vi "EditorPDF setPDFList.vi"(8 "error in (no error)":errorcluster, 11 "CreatePDF in":refnum<class "CreatePDF.lvclass">) -> (0 "error out":errorcluster, 3 "CreatePDF out":refnum<class "CreatePDF.lvclass">)   [LabVIEW 2018, in "CreatePDF.lvclass"]
uses:
  CreatePDF.lvclass
  <vilib>/Simplicity AI/SAI_PDF_API/Classes/Context/Controls/SAI_PDF_Text Align.ctl
  <vilib>/Simplicity AI/SAI_PDF_API/Classes/Context/Controls/SAI_PDF_Table Settings.ctl
  <vilib>/Simplicity AI/SAI_PDF_API/Classes/Context/Controls/SAI_PDF_Table Parameters.ctl
  <vilib>/Simplicity AI/SAI_PDF_API/Classes/Table Builder/Controls/SAI_PDF_Table Cell Alignment.ctl
  <vilib>/Simplicity AI/SAI_PDF_API/Classes/Context/Controls/SAI_PDF_Vertical Align.ctl
  CreatePDF.lvclass/CreatePDF.ctl
  <vilib>/Simplicity AI/SAI_PDF_API/Classes/Context/Methods/Public/Low Level/Add/SAI_PDF_Add Paragraph.vi
  <vilib>/Simplicity AI/SAI_PDF_API/Classes/Context/Context.lvclass
  <vilib>/Simplicity AI/SAI_PDF_API/Classes/Table Builder/Table Builder.lvclass
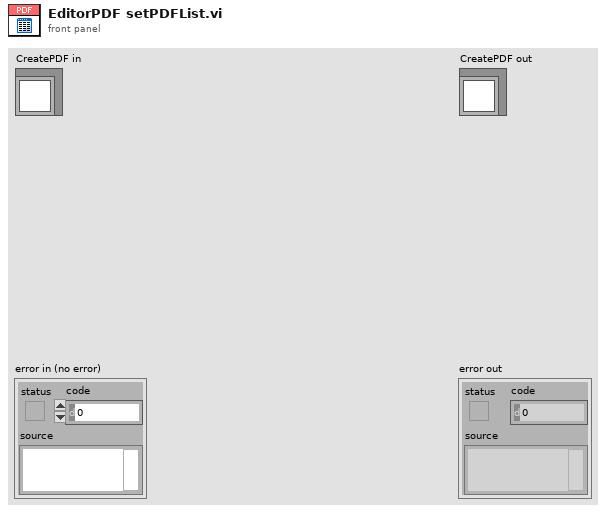
[diagram p1: front panel]
types:
  T1 = typedef "SAI_PDF_Toolkit.lvlib/Context.lvclass/SAI_PDF_Table Settings.ctl" = cluster{"Column Widths":sgl[], "Parameters":T2, "Cell Alignment":T3}
  T2 = typedef "SAI_PDF_Toolkit.lvlib/Context.lvclass/SAI_PDF_Table Parameters.ctl" = cluster{"Show Header":bool, "Background Colour":u32, "Colour Alternate Lines":bool, "Min Row Height":sgl, "Border Width":sgl}
  T3 = typedef "SAI_PDF_Toolkit.lvlib/Table Builder.lvclass/SAI_PDF_Table Cell Alignment.ctl" = cluster{"Horizontal Align":T4, "Vertical Align":T5}
  T4 = typedef "SAI_PDF_Toolkit.lvlib/Context.lvclass/SAI_PDF_Text Align.ctl" = i32
  T5 = typedef "SAI_PDF_Toolkit.lvlib/Context.lvclass/SAI_PDF_Vertical Align.ctl" = i32
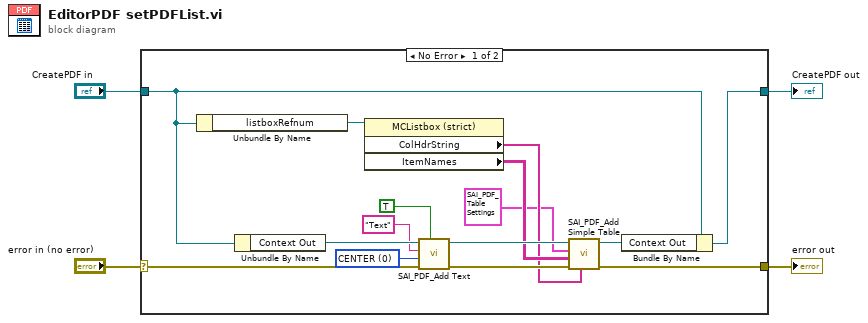
[diagram p0: block diagram]
diagram:
  n1 = case shown="No Error" "error in (no error)" {
    selector: "error in (no error)" -> [w15 w21]
    tunnel: [w9 w21] -> w3
    tunnel: [w6 w20] -> w1
    tunnel: "CreatePDF in" -> [w8 w20]
    frame No Error {
      w19 = T4 0 items=["CENTER", "JUSTIFIED", "JUSTIFIED_ALL", "LEFT", "RIGHT"] ("Align")
      n2 = Unbundle By Name(w8) -> ("listboxRefnum"=w17:refnum<vi>)
      n3 = Unbundle By Name(w8) -> ("Context Out"=w16:refnum<class "Context.lvclass">)
      n4 = property class="MCListbox (strict)"(reference=w17) -> ("ColHdrString"=w11:string[], "ItemNames"=w12:string[][])  [unwired: 1 in, 2 out]
      n5 = call-poly <vilib>:"SAI_PDF_Add Text.vi"("Add Line Feeds (F:No)"=TRUE, "error in"=w15, "Align (Left)"=w19, "Text"="Text", "Context In"=w16) -> ("error out"=w13:errorcluster, "Context Out"=w14:refnum<class "Context.lvclass">)  [unwired: 5 out]
      n6 = call <vilib>:"SAI_PDF_Add Simple Table.vi"("Headers"=w11, "error in"=w13, "Data"=w12, "Table Settings"=T1 {"Column Widths"=[], "Parameters"={"Show Header"=TRUE, "Background Colour"=14474460, "Colour Alternate Lines"=TRUE, "Min Row Height"=15.0, "Border Width"=0.0}, "Cell Alignment"={"Horizontal Align"=0, "Vertical Align"=2}}, "Context In"=w14) -> ("error out"=w9:errorcluster, "Context Out"=w7:refnum<class "Context.lvclass">)  [unwired: 1 in, 4 out]
      n7 = Bundle By Name(cluster=w8, "Context Out"=w7) -> (w6:refnum<class "CreatePDF.lvclass">)
    }
    frame Error {
    }
  }
  "error out" <- w3
  "CreatePDF out" <- w1
